vi "BruteForcer.vi"(10 "Index":i32, 11 "Array in":u8[](array[numeric])) -> (2 "Rolled Over?":bool, 3 "Array out":u8[](array[numeric]))   [LabVIEW 2022 SP3]
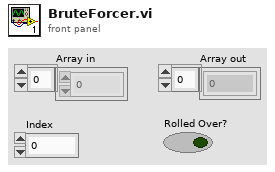
[diagram p1: front panel]
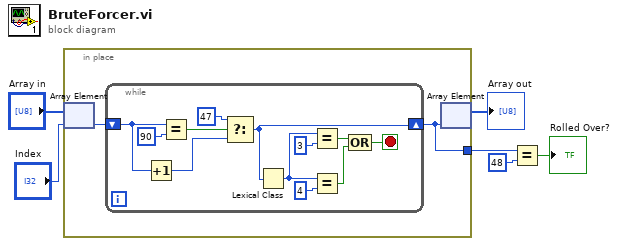
[diagram p0: block diagram]
diagram:
  n1 = in-place {
    in-place-border: [w7] -> w5
    n2 = in-place-array #1("Array in", "Index") -> (w8:u8)
    n3 = while {
      shift-right: [w9] -> w7
      shift-left: w8 -> [w13]
      stop <- w15 stop-if-true
      n4 = Increment(x=w13) -> (x+1=w10:u8)
      n5 = Equal?(x=w13, y=u8 90) -> (x = y?=w12:bool)
      n6 = Select(t=u8 47, s=w12, f=w10) -> (s? t:f=w9:u8)
      n7 = Lexical Class(1:w9) -> (0:w20:i16)
      n8 = Equal?(x=w20, y=i16 3) -> (x = y?=w16:bool)
      n9 = Equal?(x=w20, y=i16 4) -> (x = y?=w17:bool)
      n10 = Compound Arithmetic op=OR(w16, w17) -> (w15:bool)
    }
    n11 = in-place-array #1(w7) -> (→"Array out":u8[])  [unwired: 1 out]
  }
  n12 = Equal?(x=w5, y=u8 48) -> (x = y?=→"Rolled Over?":bool)
